vi "KepcoDCPwr Configure Trigger Source [TRG].vi"(0 "VISA Session":refnum<visa-resource-name>, 5 "Model In":string, 7 "channel name (\"\")":string="\"\"", 9 "Trigger Source":enum16{"BUS", "External", "Immediate"}(ring), 11 "error in (no error)":errorcluster {"code" format="%.0x"}) -> (4 "VISA Session Out":refnum<visa-resource-name>, 6 "Model Out":string, 8 "channel name out (\"\")":string="\"\"" caption="channel name Out (\"\")", 15 "error out":errorcluster {"code" format="%.0x"})   [LabVIEW 2010]
doc: "Configures the trigger source the power supply waits for before changing the output signal. When the power supply receives a trigger signal on the source you specify, it changes its current limit and voltage level values."
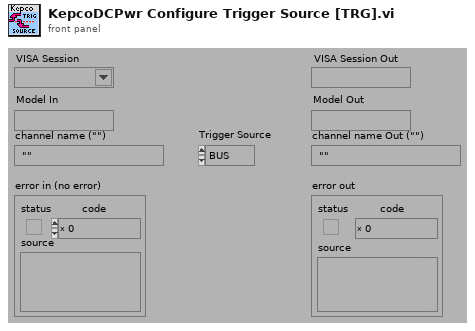
[diagram p1: front panel]
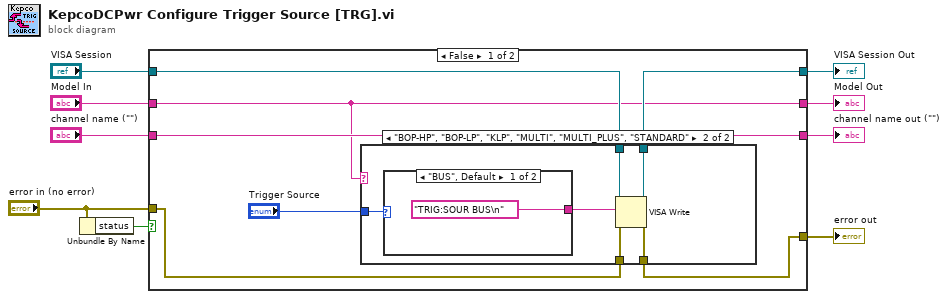
[diagram p0: block diagram]
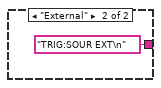
[diagram p3: hidden frame]
diagram:
  n1 = Unbundle By Name("error in (no error)") -> ("status"=w8:bool)
  n2 = case shown="False" w8 {
    tunnel: [w12 w30] -> w9
    tunnel: "error in (no error)" -> [w13 w30]
    tunnel: "VISA Session" -> [w15 w29]
    tunnel: [w14 w29] -> w3
    tunnel: "Model In" -> [w10 w28]
    tunnel: [w10 w28] -> w2
    tunnel: "channel name (\"\")" -> [w16 w27]
    tunnel: [w16 w27] -> w1
    frame False {
      n3 = case shown="\"BOP-HP\", \"BOP-LP\", \"KLP\", \"MULTI\", \"MULTI_PLUS\", \"STANDARD\"" w10 {
        tunnel: w13 -> [w18 w24]
        tunnel: [w18 w23] -> w12
        tunnel: w15 -> [w17 w22]
        tunnel: [w17 w21] -> w14
        tunnel: "Trigger Source" -> [_ w19]
        frame "", Default {
        }
        frame "BOP-HP", "BOP-LP", "KLP", "MULTI", "MULTI_PLUS", "STANDARD" {
          n4 = case shown="\"BUS\", Default" w19 {
            tunnel: ["TRIG:SOUR BUS\n" "TRIG:SOUR EXT\n"] -> w20
            frame "BUS", Default {
            }
            frame "External" {
            }
          }
          n5 = VISA Write(VISA resource name=w22, write buffer=w20, error in (no error)=w24) -> (VISA resource name out=w21:refnum<visa-resource-name>, error out=w23:errorcluster)  [unwired: 1 out]
        }
      }
    }
    frame True {
    }
  }
  "error out" <- w9
  "channel name out (\"\")" <- w1
  "Model Out" <- w2
  "VISA Session Out" <- w3
